vi "Read Max readings.vi"(8 "error in (no error)":errorcluster, 11 "Keithley 622x2182 Driver in":refnum<class "Keithley 622x2182 Driver.lvclass">) -> (0 "error out":errorcluster, 2 "Max readings":string="INF", 3 "Keithley 622x2182 Driver out":refnum<class "Keithley 622x2182 Driver.lvclass">)   [LabVIEW 2021, in "Keithley 622x2182 Driver.lvclass"]
uses:
  Keithley 622x2182 Driver.lvclass
  Keithley 622x2182 Driver.lvclass/Keithley 622x2182 Driver.ctl
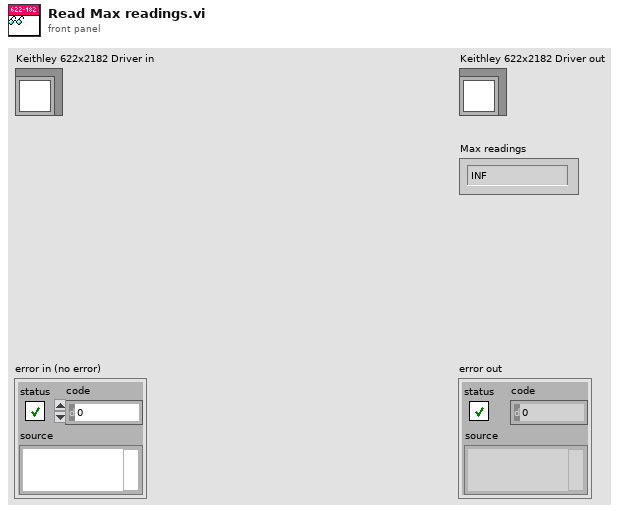
[diagram p1: front panel]
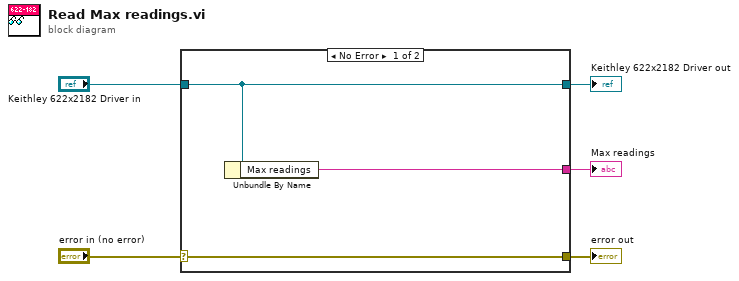
[diagram p0: block diagram]
diagram:
  n1 = case shown="No Error" "error in (no error)" {
    selector: "error in (no error)" -> [w8 w9]
    tunnel: [w8 w9] -> w4
    tunnel: [w7 w10] -> w2
    tunnel: "Keithley 622x2182 Driver in" -> [w7 w10]
    tunnel: [w6 _] -> w1
    frame No Error {
      n2 = Unbundle By Name(w7) -> ("Max readings"=w6:string)
    }
    frame Error {
    }
  }
  "error out" <- w4
  "Keithley 622x2182 Driver out" <- w2
  "Max readings" <- w1
